vi "Receiver.vi"() -> ()   [LabVIEW 2022 SP3]
doc: "Use this template to build a producer/consumer design pattern. Use this template when you need to execute a process, such as data analysis, when a data source, such as a triggered acquisition, produces data at an uneven rate and you need to execute the process when the data becomes available."
uses:
  ButtonStates.ctl
  <vilib>/MakerHub/LINX/Public/Utilities/Open Serial.vi
  <vilib>/MakerHub/LINX/LMH-LINX.lvlib
panel:
  out "Morse Code Received":string
  out "Current Morse Reading":string
  in  "Pulse Interval (ms)":u32=10
  out "Rise Time (ms)":u32
  out "Fall Time (ms)":u32
  out "Falling Edge (absolute)":u32
  out "Rise Edge (absolute)":u32
  in  "stop":bool
  out "Morse Code Translated":string
  out "Total Error Out":errorcluster
  in  "PhotoResistor Pin":u8
  out "Pulse Width":dbl(graph)
  out "Rising Edge Detection":i32(graph)
  out "Falling Edge Detection":i32(graph)
  out "Time":u32
  in  "Serial Port":refnum<visa-resource-name>="N/A"
  # "RECEIVE MORSE CODE"
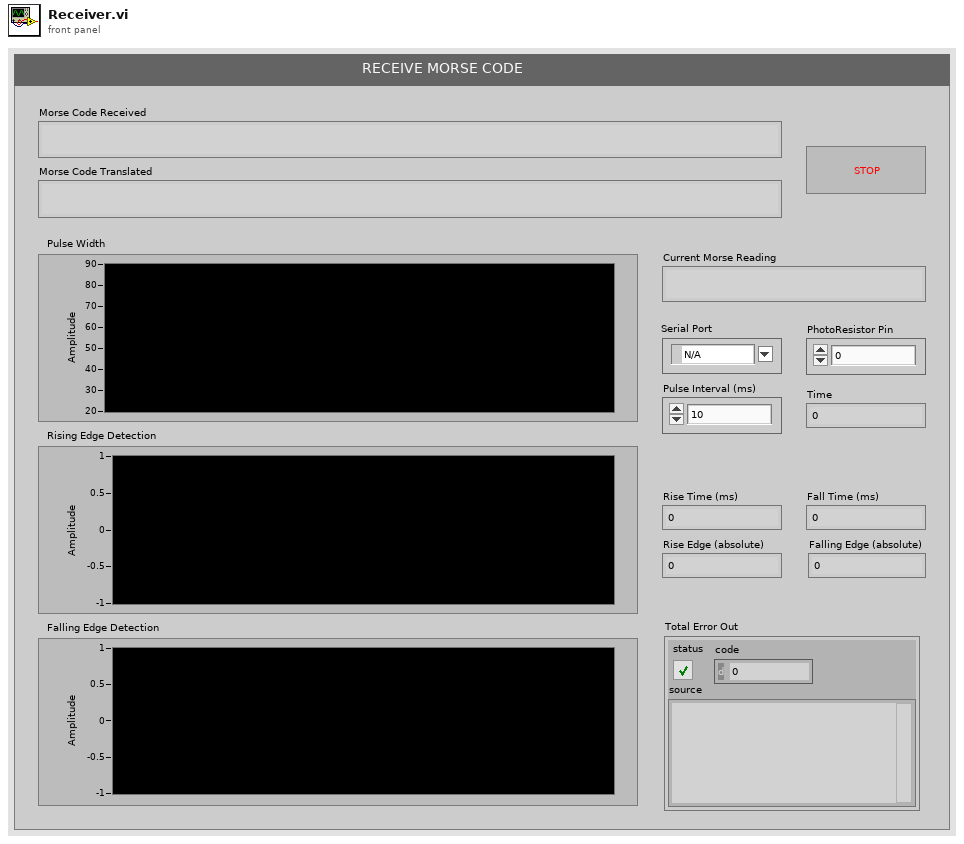
[diagram p1: front panel]
types:
  T1 = typedef "ButtonStates.ctl" = enum16{"Rising", "Just After Rising", "Falling", "Just After Falling", "Default"}
  T2 = typedef "LMH-LINX.lvlib/LINX Ref.ctl" = cluster{"IO":T3, "Interface":T4, "LINX Device Config":T5}
  T3 = typedef "LMH-LINX.lvlib/Platform.ctl" = enum16{"Remote", "Local"}
  T4 = typedef "LMH-LINX.lvlib/Interface.ctl" = enum16{"Serial", "TCP"}
  T5 = typedef "LMH-LINX.lvlib/Device.lvlib/LINX Device Config.ctl" = cluster{"Interface":T4, "COM Port":refnum<visa-resource-name>, "TCP Configuration":T6, "Device Family":u8, "Device ID":u8, "Device Name":string, "TCP Ref":refnum<k5>, "Channels":T7}
  T6 = typedef "LMH-LINX.lvlib/Device.lvlib/TCP Config.ctl" = cluster{"IP Address":string, "Port":u16}
  T7 = typedef "LMH-LINX.lvlib/Channels.ctl" = cluster{"DI":u8[], "DO":u8[], "AI":u8[], "AO":u8[], "PWM":u8[], "QE":u8[], "UART":u8[], "I2C 2":u8[], "SPI":u8[], "CAN":u8[], "Servo":u8[], "AI Ref (V)":dbl, "AI Resolution (Bits)":u8, "AO Ref (V)":dbl, "AO Resolution (Bits)":u8}
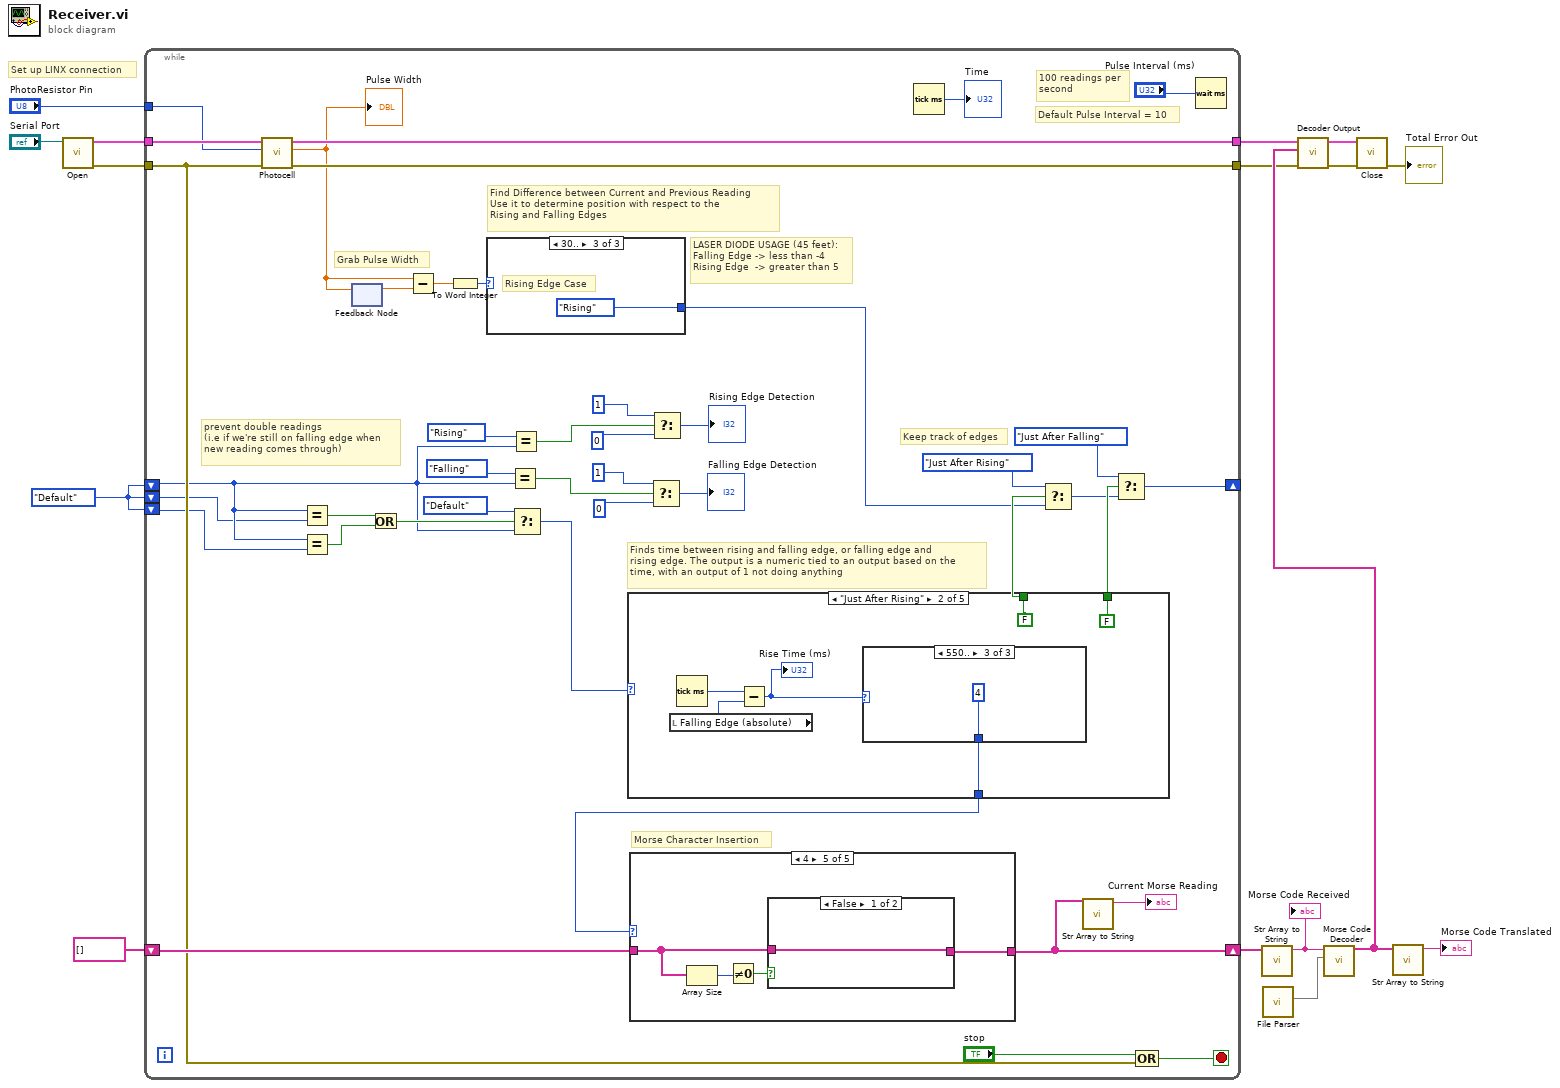
[diagram p0: block diagram]
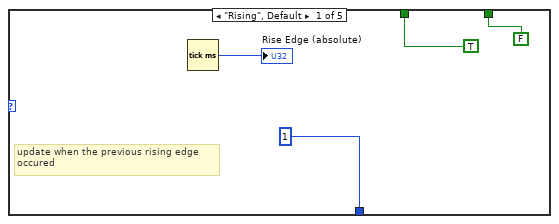
[diagram p2: hidden frame]
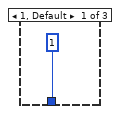
[diagram p3: hidden frame]
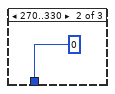
[diagram p4: hidden frame]
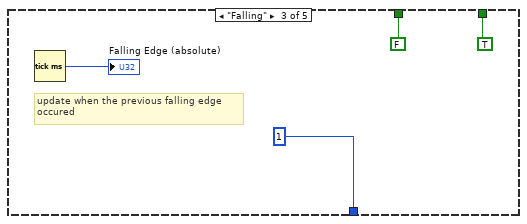
[diagram p5: hidden frame]
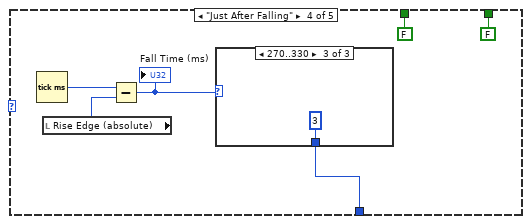
[diagram p6: hidden frame]
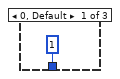
[diagram p7: hidden frame]
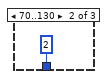
[diagram p8: hidden frame]
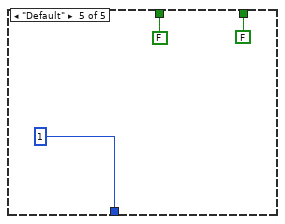
[diagram p9: hidden frame]
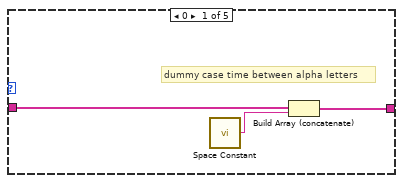
[diagram p10: hidden frame]
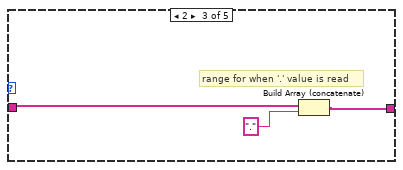
[diagram p12: hidden frame]
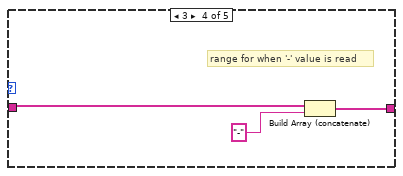
[diagram p13: hidden frame]
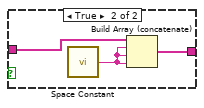
[diagram p14: hidden frame]
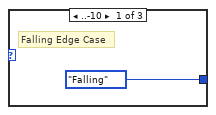
[diagram p15: hidden frame]
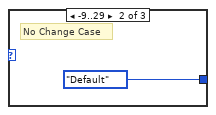
[diagram p16: hidden frame]
diagram:
  w2 = ButtonStates."Default"
  # "Set up LINX connection"
  n1 = call-poly <vilib>:"Open.vi"("Serial Port"="Serial Port") -> ("Error Out"=w12:errorcluster, "LINX Resource"=w11:T2)  [unwired: 8 in, 1 out]
  n2 = while {
    shift-right: [w23] -> _
    shift-left: w2 -> [w22]
    tunnel: w11 -> [w54]
    tunnel: w12 -> [w37]
    tunnel: [w53] -> w5
    tunnel: [w52] -> w6
    shift-right: [w20] -> w10
    shift-left: string[] [] -> [w43]
    shift-left: w2 -> [w18]
    tunnel: "PhotoResistor Pin" -> [w39]
    shift-left: w2 -> [w17]
    stop <- w36 stop-if-true
    # "Morse Character Insertion"
    # "Finds time between rising and falling edge, or falling edge and \nrising edge. The output is a numeric tied to an output based on the \ntime, with an output of 1 not doing anything"
    # "Find Difference between Current and Previous Reading\nUse it to determine position with respect to the \nRising and Falling Edges"
    # "Keep track of edges"
    # "Grab Pulse Width"
    # "LASER DIODE USAGE (45 feet):\nFalling Edge -> less than -4\nRising Edge  -> greater than 5"
    # "Default Pulse Interval = 10"
    # "prevent double readings \n(i.e if we're still on falling edge when \nnew reading comes through)"
    # "100 readings per \nsecond"
    n3 = call <vilib>:"Photocell.vi"("Error In"=w37, "AI Channel"=w39, "LINX Resource"=w54) -> ("Error Out"=w52:errorcluster, "Value (0-100)"=w50:dbl, "LINX Resource"=w53:T2)  [unwired: 6 in]
    "Pulse Width" <- w50
    n4 = Equal?(x=w22, y=w18) -> (x = y?=w33:bool)
    n5 = Equal?(x=w22, y=w17) -> (x = y?=w34:bool)
    n6 = feedback-in #1(w50) -> ()
    n7 = feedback #1() -> (w58:dbl)  [unwired: 1 in]
    n8 = Or(x=w33, y=w34) -> (x .or. y?=w32:bool)
    n9 = Subtract(x=w50, y=w58) -> (x-y=w51:dbl)
    n10 = To Word Integer(number=w51) -> (16bit integer=w57:i16)
    n11 = case shown="30.." w57 {
      tunnel: [ButtonStates."Falling" ButtonStates."Default" ButtonStates."Rising"] -> w28
      frame ..-10 {
        # "Falling Edge Case"
      }
      frame -9..29 {
        # "No Change Case"
      }
      frame 30.. {
        # "Rising Edge Case"
      }
    }
    n12 = Equal?(x=ButtonStates."Falling", y=w22) -> (x = y?=w45:bool)
    n13 = Equal?(x=ButtonStates."Rising", y=w22) -> (x = y?=w49:bool)
    n14 = Select(t=ButtonStates."Default" ("x"), s=w32, f=w22) -> (s? t:f=w30:T1)
    n15 = case shown="\"Just After Rising\"" w30 {
      tunnel: [u32 1 w67 u32 1 w79 u32 1] -> w35
      tunnel: [TRUE FALSE FALSE FALSE FALSE] -> w29
      tunnel: [FALSE FALSE TRUE FALSE FALSE] -> w26
      frame "Rising", Default {
        # "update when the previous rising edge \noccured"
        n16 = Tick Count (ms)() -> (millisecond timer value=→"Rise Edge (absolute)":u32)
      }
      frame "Just After Rising" {
        n17 = local read "Falling Edge (absolute)"() -> (w65:u32)
        n18 = Tick Count (ms)() -> (millisecond timer value=w68:u32)
        n19 = Subtract(x=w68, y=w65) -> (x-y=w66:u32)
        "Rise Time (ms)" <- w66
        n20 = case shown="550.." w66 {
          tunnel: [u32 1 u32 0 u32 4] -> w67
          frame 1, Default {
          }
          frame 270..330 {
          }
          frame 550.. {
          }
        }
      }
      frame "Falling" {
        # "update when the previous falling edge \noccured"
        n21 = Tick Count (ms)() -> (millisecond timer value=→"Falling Edge (absolute)":u32)
      }
      frame "Just After Falling" {
        n22 = Tick Count (ms)() -> (millisecond timer value=w81:u32)
        n23 = local read "Rise Edge (absolute)"() -> (w78:u32)
        n24 = Subtract(x=w81, y=w78) -> (x-y=w80:u32)
        "Fall Time (ms)" <- w80
        n25 = case shown="270..330" w80 {
          tunnel: [u32 1 u32 2 u32 3] -> w79
          frame 0, Default {
          }
          frame 70..130 {
          }
          frame 270..330 {
          }
        }
      }
      frame "Default" {
      }
    }
    n26 = case shown="4" w35 {
      tunnel: [w89 w91 w92 w95 w101] -> w20
      tunnel: w43 -> [w88 w91 w93 w96 w100]
      frame 0 {
        # "dummy case time between alpha letters"
        n27 = call <vilib>:"Space Constant.vi"() -> ("String"=w90:string)
        n28 = Build Array (concatenate)(w88, w90) -> (w89:string[])
      }
      frame 1, Default {
        # "1) allows for delay between morse chars  w/o\nappending string array\n2) after morse char is read, prevents additional \nchars from being read"
      }
      frame 2 {
        # "range for when '.' value is read"
        n29 = Build Array (concatenate)(w93, ".") -> (w92:string[])
      }
      frame 3 {
        # "range for when '-' value is read"
        n30 = Build Array (concatenate)(w96, "-") -> (w95:string[])
      }
      frame 4 {
        n31 = Array Size(array=w100) -> (size(s)=w99:i32)
        n32 = Not Equal To 0?(x=w99) -> (x != 0?=w98:bool)
        n33 = case shown="False" w98 {
          tunnel: w100 -> [w102 w105]
          tunnel: [w102 w103] -> w101
          frame False {
          }
          frame True {
            n34 = call <vilib>:"Space Constant.vi"() -> ("String"=w104:string)
            n35 = Build Array (concatenate)(w105, w104, w104, w104) -> (w103:string[])
          }
        }
      }
    }
    n36 = Select(t=1, s=w45, f=0) -> (s? t:f=→"Falling Edge Detection":i32)
    n37 = Select(t=1, s=w49, f=0) -> (s? t:f=→"Rising Edge Detection":i32)
    n38 = Tick Count (ms)() -> (millisecond timer value=→"Time":u32)
    n39 = Select(t=ButtonStates."Just After Rising", s=w29, f=w28) -> (s? t:f=w24:T1)
    n40 = call "Str Array to String.vi"("Array"=w20) -> ("String"=→"Current Morse Reading":string)  [unwired: 10 in]
    n41 = Select(t=ButtonStates."Just After Falling", s=w26, f=w24) -> (s? t:f=w23:T1)
    n42 = Compound Arithmetic op=OR("stop", w37) -> (w36:bool)
    n43 = Wait (ms)(milliseconds to wait="Pulse Interval (ms)") -> ()  [unwired: 1 out]
  }
  n44 = call "Str Array to String.vi"("Array"=w10) -> ("String"=w9:string)  [unwired: 10 in]
  "Morse Code Received" <- w9
  n45 = call "File Parser.vi"() -> ("Morse-Letter Map (output 2)"=w1:map{string, string})  [unwired: 9 in, 2 out]
  n46 = call "Morse Code Decoder.vi"("Map"=w1, "Message to Decode"=w9) -> ("Decoded Array"=w7:string[])  [unwired: 8 in, 1 out]
  n47 = call "Decoder Output.vi"("Error In"=w6, "Decoded Array"=w7, "LINX Resource"=w5) -> ("Error Out"=w3:errorcluster, "LINX Resource (Out)"=w4:T2)  [unwired: 7 in]
  n48 = call <vilib>:"Close.vi"("Error In"=w3, "LINX Resource"=w4) -> ("Error Out"=→"Total Error Out":errorcluster)  [unwired: 9 in]
  n49 = call "Str Array to String.vi"("Array"=w7) -> ("String"=→"Morse Code Translated":string)  [unwired: 10 in]
